vi "Stop Helper Loops.vi"(8 "error in (no error)":errorcluster, 11 "Helper Loop In":refnum<class "Helper Loop.lvclass">) -> (0 "error out":errorcluster, 3 "Helper Loop Out":refnum<class "Helper Loop.lvclass">)   [LabVIEW 2020, in "Helper Loop.lvclass"]
doc: "This method stops the helper loop.The Helper Action may stop the helper loop by throwing an error. If this has happened prior to calling this method, a time out will occur."
uses:
  Helper Loop.lvclass
  Process/Process.lvclass
  Process/Process.lvclass/Process.ctl
  <vilib>/Utility/error.llb/Clear Errors.vi
  Broadcast Event Helpers/Execution timer.vi
  <vilib>/Utility/error.llb/Error Cluster From Error Code.vi
  Broadcast Event Helpers/Dequeue Broadcast Message.vi
  <vilib>/ErrorRing/Error Ring.xnode
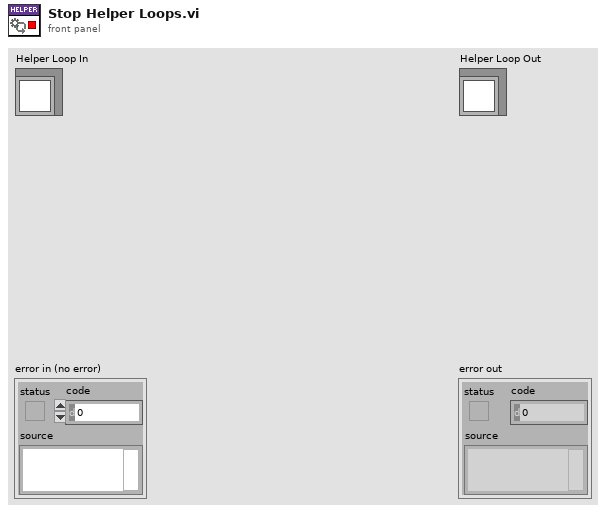
[diagram p1: front panel]
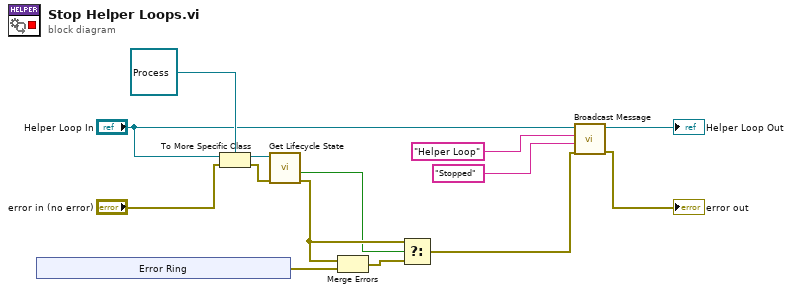
[diagram p0: block diagram]
diagram:
  n1 = xnode "Error Ring"() -> ("error out"=w7:errorcluster)
  n2 = To More Specific Class(target class=refnum<class "Process.lvclass"> refnum ("Process Out"), reference="Helper Loop In", error in="error in (no error)") -> (specific class reference=w13:refnum<class "Process.lvclass">, error out=w11:errorcluster)
  n3 = call "Get Lifecycle State.vi"("error in (no error)"=w11, "Process In"=w13) -> ("error out"=w10:errorcluster, "In Process Loop?"=w9:bool)  [unwired: 6 in, 2 out]
  n4 = Merge Errors(w10, w7) -> (w8:errorcluster)
  n5 = Select(t=w10, s=w9, f=w8) -> (s? t:f=w3:errorcluster)
  n6 = call-dynamic "Broadcast Message.vi"("error in (no error)"=w3, "Message Data"="Stopped" ("Message"), "Message"="Helper Loop", "Helper Loop in"="Helper Loop In") -> ("error out"=→"error out":errorcluster, "Helper Loop out"=→"Helper Loop Out":refnum<class "Helper Loop.lvclass">)  [unwired: 6 in]
